vi "Configure Arbitrary Waveform.vi"(0 "VISA resource name":refnum<visa-resource-name>, 1 "Arbitrary Waveform Name":string, 2 "Draw Arbitrary Waveform":u16(ring) items=["Arbitrary Waveform Line", "Arbitrary Waveform Point"], 3 "Point Address":dbl, 4 "Point Data":dbl min=-2048.0 max=2047.0, 5 "error in (no error)":errorcluster, 6 "Line Start Address":dbl, 7 "Stop Data":dbl, 8 "Line Stop Address":dbl, 9 "Start Data":dbl min=-2048.0 max=2047.0, 10 "Arbitrary Waveform Amplitude (1.0 Vpp)":dbl=1.0, 11 "Arbitrary Waveform Amplitude Units":u16(ring) items=["Vpp", "Vrms", "dBm"], 12 "Arbitrary Waveform Frequency (1000 Hz)":dbl=1000.0, 13 "Arbitrary Waveform DC Offset (0.00 V)":dbl) -> (14 "VISA resource name out":refnum<visa-resource-name>, 19 "error out":errorcluster)   [LabVIEW 2015, in "Fluke 28x Series.lvlib"]
doc: "Sets the waveform parameters for an existing arbitrary waveform and make it the active waveform function. This VI should be called after the Create Arbitrary Waveform VI."
uses:
  <instrlib>/Fluke 28x Series/Fluke 28x Series.lvlib
panel:
  # "Draw Arbitrary Waveform Point"
  # "Draw Arbitrary Waveform Line"
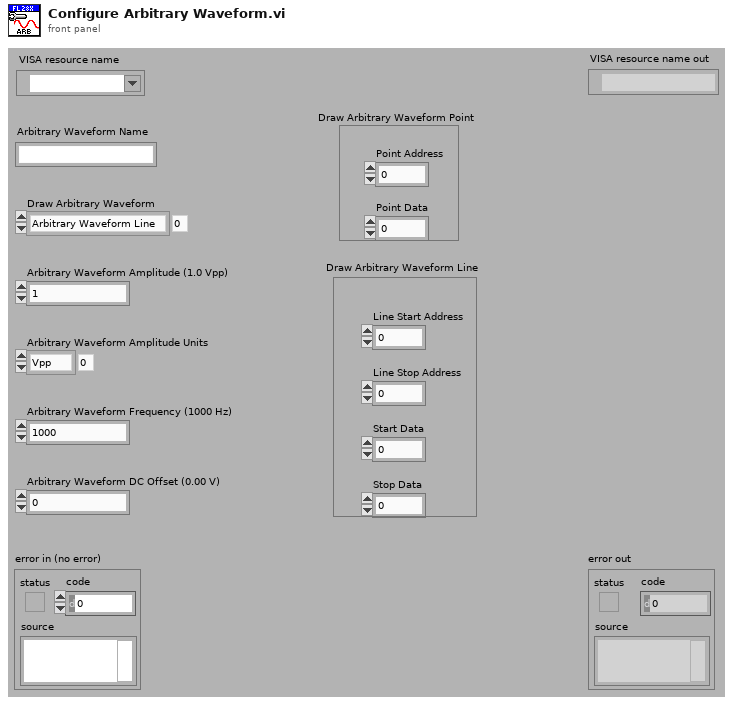
[diagram p1: front panel]
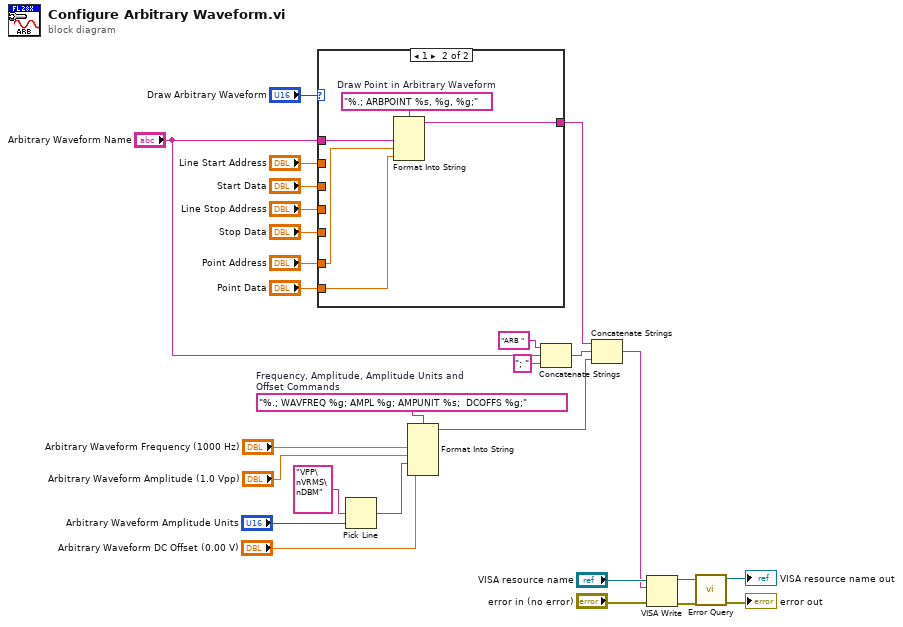
[diagram p0: block diagram]
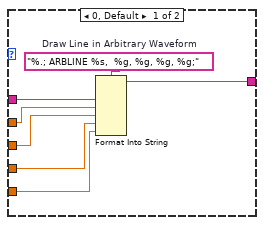
[diagram p2: hidden frame]
diagram:
  w9 = "%.; WAVFREQ %g; AMPL %g; AMPUNIT %s;  DCOFFS %g;"  # Frequency, Amplitude, Amplitude Units and Offset Commands
  n1 = case shown="1" "Draw Arbitrary Waveform" {
    tunnel: "Arbitrary Waveform Name" -> [w33 w38]
    tunnel: "Line Start Address" -> [w32 _]
    tunnel: "Start Data" -> [w31 _]
    tunnel: "Line Stop Address" -> [w29 _]
    tunnel: "Stop Data" -> [w30 _]
    tunnel: "Point Address" -> [_ w37]
    tunnel: "Point Data" -> [_ w36]
    tunnel: [w28 w35] -> w11
    frame 0, Default {
      w34 = "%.; ARBLINE %s,  %g, %g, %g, %g;"  # Draw Line in Arbitrary Waveform
      n2 = Format Into String(format string=w34, w33, w32, w31, w29, w30) -> (resulting string=w28:string)  [unwired: 2 in, 1 out]
    }
    frame 1 {
      w39 = "%.; ARBPOINT %s, %g, %g;"  # Draw Point in Arbitrary Waveform
      n3 = Format Into String(format string=w39, w38, w37, w36) -> (resulting string=w35:string)  [unwired: 2 in, 1 out]
    }
  }
  n4 = Pick Line(multi-line string="VPP\nVRMS\nDBM", line index="Arbitrary Waveform Amplitude Units") -> (output string=w4:string)  [unwired: 1 in]
  n5 = Format Into String(format string=w9, "Arbitrary Waveform Frequency (1000 Hz)", "Arbitrary Waveform Amplitude (1.0 Vpp)", w4, "Arbitrary Waveform DC Offset (0.00 V)") -> (resulting string=w2:string)  [unwired: 2 in, 1 out]
  n6 = Concatenate Strings("ARB " ("string"), "Arbitrary Waveform Name", "; " ("string")) -> (w12:string)
  n7 = Concatenate Strings(w11, w12, w2) -> (w10:string)
  n8 = VISA Write(VISA resource name="VISA resource name", write buffer=w10, error in (no error)="error in (no error)") -> (VISA resource name out=w27:refnum<visa-resource-name>, error out=w26:errorcluster)  [unwired: 1 out]
  n9 = call <instrlib>:"Error Query.vi"("error in (no error)"=w26, "VISA resource name"=w27) -> ("error out"=→"error out":errorcluster, "VISA resource name out"=→"VISA resource name out":refnum<visa-resource-name>)  [unwired: 6 in, 2 out]
